vi "FVIR_LDO_Agilent_34972A.vi"(8 "error in":errorcluster, 10 "VISA Refnum in":refnum<visa-resource-name>, 11 "Message Queues":T1) -> (0 "error out":errorcluster)   [LabVIEW 2020]
uses:
  Message Queue/All Message Queues.ctl
  Message Queue/Message Cluster.ctl
  Agilent Data.ctl
  Message Queue/Enqueue Message (Single).vi
  Message Queue/Message Queue.lvlib
  Drivers/Agilent 34972/Agilent 34970.lvlib
panel:
  out "Loop Count":i32
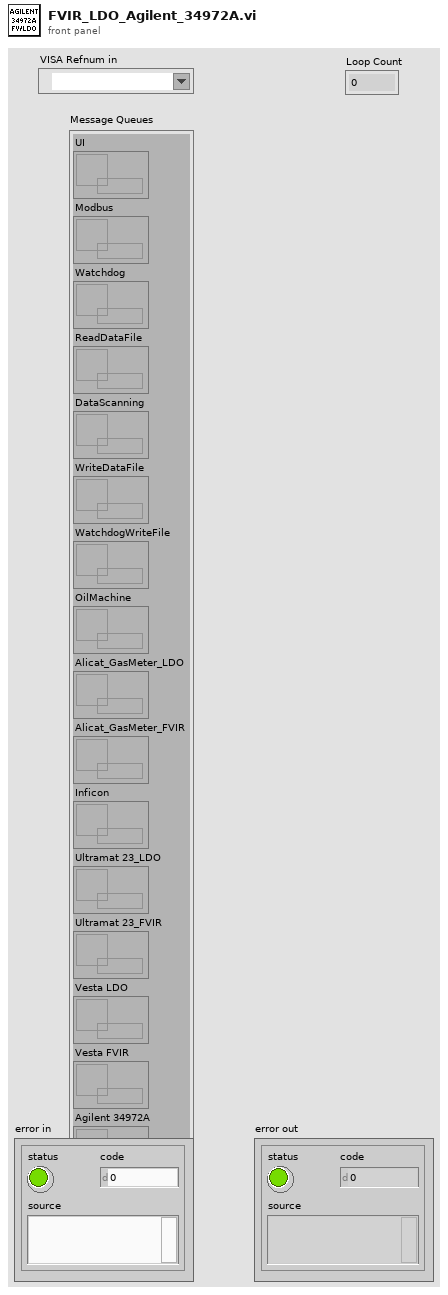
[diagram p1: front panel]
types:
  T1 = typedef "Message Queue.lvlib/All Message Queues.ctl" = cluster{"UI":refnum<queue>, "Modbus":refnum<queue>, "Watchdog":refnum<queue>, "ReadDataFile":refnum<queue>, "DataScanning":refnum<queue>, "WriteDataFile":refnum<queue>, "WatchdogWriteFile":refnum<queue>, "OilMachine":refnum<queue>, "Alicat_GasMeter_LDO":refnum<queue>, "Inficon":refnum<queue>, "Ultramat 23_LDO":refnum<queue>, "Alicat_GasMeter_FVIR":refnum<queue>, "Ultramat 23_FVIR":refnum<queue>, "Vesta LDO":refnum<queue>, "Vesta FVIR":refnum<queue>, "Agilent 34972A":refnum<queue>}
  T2 = enum16{"100 Ohm", "1 kOhm", "10 kOhm", "100 kOhm", "1 MOhm", "10 MOhm", "100 MOhm", "Minimum", "Maximum"}
  T3 = typedef "Agilent Data.ctl" = cluster{"Temperature (F)":dbl, "Thermistor Reading (kOhms)":dbl}
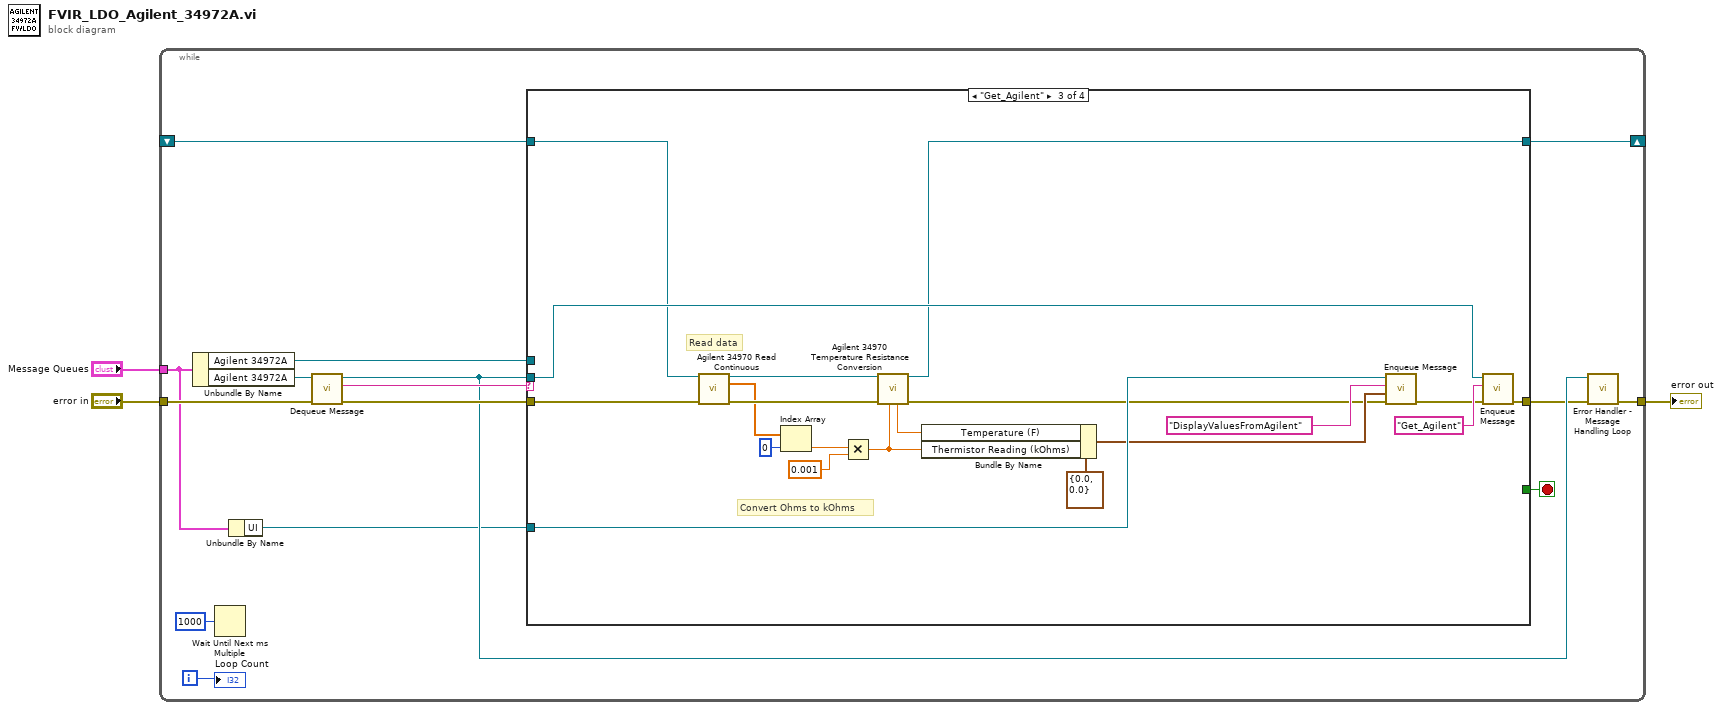
[diagram p0: block diagram]
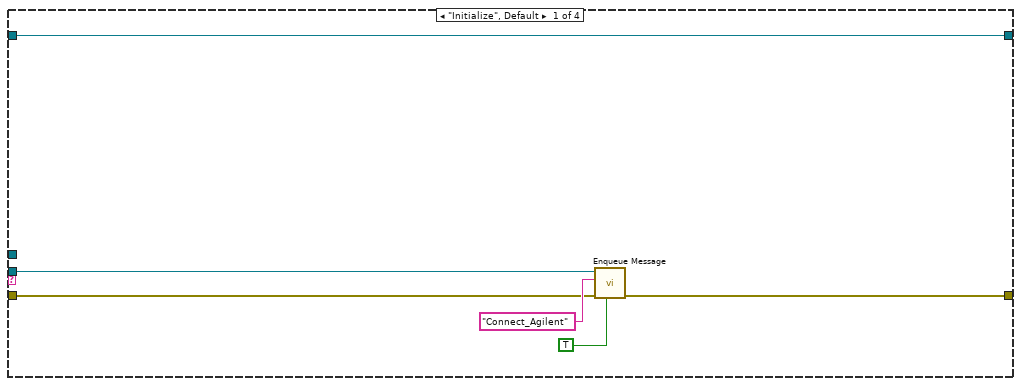
[diagram p2: hidden frame]
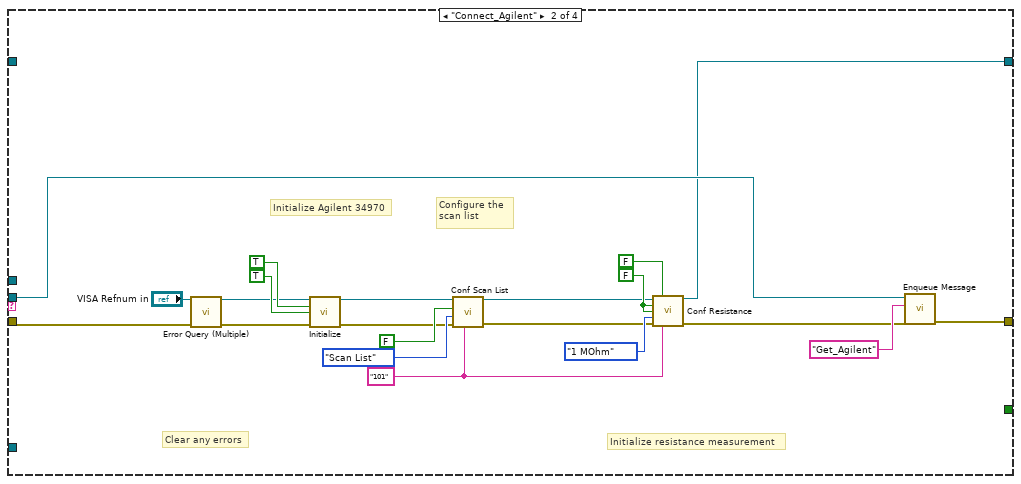
[diagram p3: hidden frame]
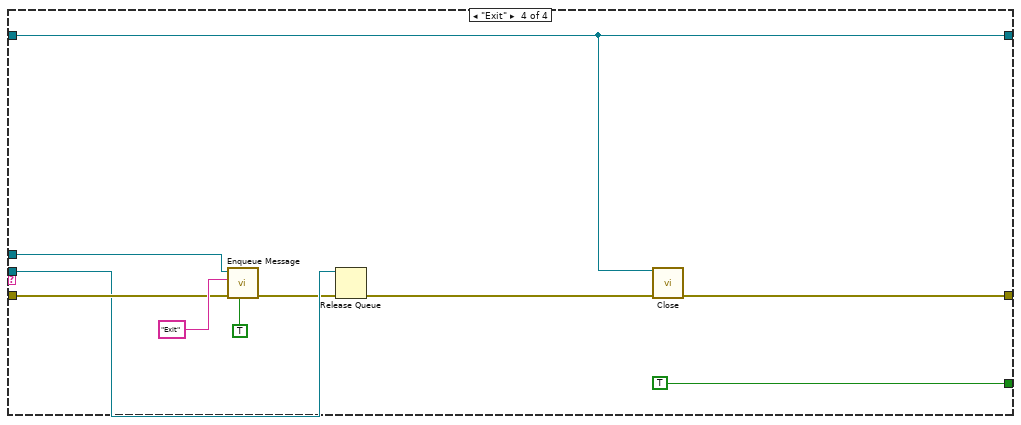
[diagram p4: hidden frame]
diagram:
  n1 = while {
    tunnel: "Message Queues" -> [w8]
    tunnel: "error in" -> [w17]
    tunnel: [w11] -> w3
    shift-right: [w6] -> _
    shift-left: _ -> [w5]
    i -> [w4]
    stop <- w14 stop-if-true
    n2 = Unbundle By Name(w8) -> ("Agilent 34972A"=w13:refnum<queue>, "Agilent 34972A"=w18:refnum<queue>)
    n3 = Wait Until Next ms Multiple(millisecond multiple=u32 1000) -> ()  [unwired: 1 out]
    n4 = Unbundle By Name(w8) -> ("UI"=w7:refnum<queue>)
    n5 = call "Dequeue Message.vi"("error in (no error)"=w17, "Message Queue"=w18) -> ("error out"=w15:errorcluster, "Message"=w16:string, "dup Message Queue"=w12:refnum<queue>)  [unwired: 6 in, 1 out]
    n6 = case shown="\"Get_Agilent\"" w16 {
      tunnel: w15 -> [w23 w25 w51 w70]
      tunnel: [w22 w44 w60 w66] -> w10
      tunnel: [_ _ _ TRUE] -> w14
      tunnel: w13 -> [_ _ _ w71]
      tunnel: w12 -> [w21 w43 w59 w69]
      tunnel: w7 -> [_ _ w63 _]
      tunnel: [w20 w26 w52 w65] -> w6
      tunnel: w5 -> [w20 _ w53 w65]
      frame "Initialize", Default {
        n7 = call-poly "Enqueue Message.vi"("Priority Message? (F)"=TRUE, "error in (no error)"=w23, "Message"="Connect_Agilent", "Message Queue"=w21) -> ("error out"=w22:errorcluster)  [unwired: 6 in, 1 out]
      }
      frame "Connect_Agilent" {
        w41 = FALSE ("4 Wire/2 Wire (F:2)")
        w37 = "101" ("Channel List (empty)")
        # "Initialize resistance measurement"
        # "Configure the\nscan list"
        # "Clear any errors"
        # "Initialize Agilent 34970"
        n8 = call "Error Query (Multiple).vi"("VISA Resource Name"="VISA Refnum in", "error in (no error)"=w25) -> ("VISA Resource Name Out"=w28:refnum<visa-resource-name>, "error out"=w29:errorcluster)  [unwired: 10 in, 2 out]
        n9 = call "Initialize.vi"("VISA Resource Name"=w28, "ID Query (T: Check)"=TRUE, "Reset (T: Reset)"=TRUE, "error in (no error)"=w29) -> ("VISA Resource Name Out"=w33:refnum<visa-resource-name>, "error out"=w34:errorcluster)  [unwired: 10 in]
        n10 = call "Conf Scan List.vi"("Scan List (empty)"=w37, "error in (no error)"=w34, "Check Parameter (0:Scan List)"=enum16{"Scan List", "Scan Size"}."Scan List", "Set/Check (F:Set)"=FALSE, "VISA Resource Name"=w33) -> ("error out"=w35:errorcluster, "VISA Resource Name Out"=w36:refnum<visa-resource-name>)  [unwired: 4 in, 1 out]
        n11 = call "Conf Resistance.vi"("VISA Resource Name"=w36, "Check/Set (F:Set)"=FALSE, "4 Wire/2 Wire (F:2)"=w41, "Autorange? (F:OFF)"=w41, "Range (8:Maximum)"=T2."1 MOhm", "error in (no error)"=w35, "Channel List (empty)"=w37) -> ("VISA Resource Name Out"=w26:refnum<visa-resource-name>, "error out"=w27:errorcluster)  [unwired: 6 in, 1 out]
        n12 = call-poly "Enqueue Message.vi"("error in (no error)"=w27, "Message"="Get_Agilent", "Message Queue"=w43) -> ("error out"=w44:errorcluster)  [unwired: 7 in, 1 out]
      }
      frame "Get_Agilent" {
        # "Convert Ohms to kOhms"
        # "Read data"
        n13 = call "Agilent 34970 Read Continuous.vi"("VISA Resource Name"=w53, "error in (no error)"=w51) -> ("VISA resource name out"=w52:refnum<visa-resource-name>, "Output Array"=w54:dbl[], "error out"=w58:errorcluster)  [unwired: 10 in, 1 out]
        n14 = Index Array(array=w54, index=0) -> (element=w56:dbl)
        n15 = Multiply(x=w56, y=0.001) -> (x*y=w48:dbl)
        n16 = call "Agilent 34970 Temperature Resistance Conversion.vi"("Resistance Value"=w48, "error in (no error)"=w58) -> ("error out"=w46:errorcluster, "Temperature (F)"=w49:dbl)  [unwired: 8 in]
        n17 = Bundle By Name(cluster=T3 {"Temperature (F)"=0.0, "Thermistor Reading (kOhms)"=0.0}, "Temperature (F)"=w49, "Thermistor Reading (kOhms)"=w48) -> (w47:T3)
        n18 = call-poly "Enqueue Message.vi"("error in (no error)"=w46, "Message Data"=w47, "Message"="DisplayValuesFromAgilent", "Message Queue"=w63) -> ("error out"=w61:errorcluster)  [unwired: 6 in, 1 out]
        n19 = call-poly "Enqueue Message.vi"("error in (no error)"=w61, "Message"="Get_Agilent", "Message Queue"=w59) -> ("error out"=w60:errorcluster)  [unwired: 7 in, 1 out]
      }
      frame "Exit" {
        n20 = call-poly "Enqueue Message.vi"("Priority Message? (F)"=TRUE, "error in (no error)"=w70, "Message"="Exit", "Message Queue"=w71) -> ("error out"=w68:errorcluster)  [unwired: 6 in, 1 out]
        n21 = Release Queue(queue=w69, error in (no error)=w68) -> (error out=w67:errorcluster)  [unwired: 1 in, 2 out]
        n22 = call "Close.vi"("VISA Resource Name"=w65, "error in (no error)"=w67) -> ("error out"=w66:errorcluster)  [unwired: 13 in]
      }
    }
    n23 = call "Error Handler - Message Handling Loop.vi"("error in (no error)"=w10, "Message Queue"=w12) -> ("dup error in"=w11:errorcluster)  [unwired: 8 in, 1 out]
    "Loop Count" <- w4
  }
  "error out" <- w3
